vi "QSM_Push Group to Queue.vi"(8 "error in (no error)":errorcluster, 10 "Group Cmds to Push":T2[](array[typedef]), 11 "QSM_Reference":T1) -> (0 "error out":errorcluster)   [LabVIEW 2014, in "TestQSM.lvlib"]
uses:
  TestQSM.lvlib
  Controls/QSM_RunStates.ctl
  Controls/QSM_Reference.ctl
  Controls/QSM_DataType.ctl
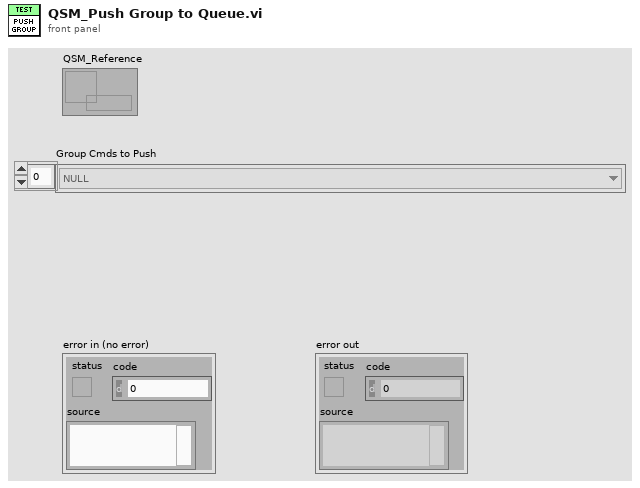
[diagram p1: front panel]
types:
  T1 = typedef "TestQSM.lvlib/QSM_Reference.ctl" = refnum<queue>
  T2 = typedef "TestQSM.lvlib/QSM_RunStates.ctl" = enum16{"NULL", "Sect01-Initialize-00-GROUP.ENQUEUE", "Sect02-Single File_Check for Parameters", "Sect02-Single File_Ask for File", "Sect02-Single File_Run Analysis", "Sect02-Single File_Write Results", "Sect03-Single ROI Calc_Check for Parameters", "Sect03-Single ROI Calc_Ask for File", "Sect03-Single ROI Calc_Run Analysis", "Sect03-Single ROI _Write Results", "Sect12-Full Dir_Check for Parameters", "Sect12-Full Dir_Ask for Dir", "Sect12-Full Dir_Check for Next Image to Process", "Sect12-Full Dir_Run Analysis", "Sect12-Full Dir_Write Results", "Sect12-Full Dir_Check if User Stopped", "Sect13-FullDir ROI Calc_Check for Parameters", "Sect13-FullDir ROI Calc_Ask for Dir", "Sect13-Full Dir ROI Calc_Check for Next Image to Process", "Sect13-Full Dir ROI Calc_Run Analysis", "Sect13-Full Dir ROI Calc_Write Results", "Sect13-Full Dir ROI Calc_Check if User Stopped", "Sect90-GUI_Config_Change UI Before Analysis", "Sect90-GUI_Config_Change UI After Analysis", "Sect90-GUI_Stop Processing Pressed", "Sect90-GUI_Stop Processing Button Set Back to F", "Sect90-GUI_Clear ROIs", "Sect99_EXIT-00-Group.Enqueue", "Sect99_EXIT-01-StopQSM"}
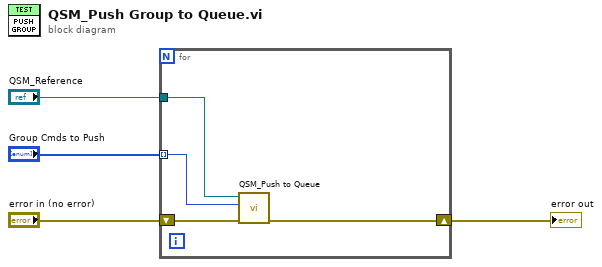
[diagram p0: block diagram]
diagram:
  n1 = for {
    tunnel: "QSM_Reference" -> [w5]
    shift-right: [w8] -> w4
    shift-left: "error in (no error)" -> [w7]
    tunnel: "Group Cmds to Push" -> [w6] mode=indexing
    n2 = call "QSM_Push to Queue.vi"("error in (no error)"=w7, "QSM_RunStates_TEST"=w6, "QSM_Reference_TEST"=w5) -> ("error out"=w8:errorcluster)  [unwired: 7 in, 1 out]
  }
  "error out" <- w4
